vi "Generate Simulated Data.vi"(7 "Type de mode":bool, 8 "error in (no error)":T2 caption="entrée d'erreur (pas d'erreur)", 9 "Péri":tag="Dev1", 10 "Longueur d'onde":dbl, 11 "Type de signal":T1) -> (0 "error out":T2 caption="sortie d'erreur", 2 "Données du graphe":waveform(dbl)[](array[waveform]))   [LabVIEW 2018, in "Acquisition.lvlib"]
doc: "Génère des exemples de waveforms en fonction du type de signal dans l'entrée Configuration du matériel."
uses:
  Acquisition.lvlib
  Signal Type.ctl
  <vilib>/Analysis/baseanly.llb/Mean (DBL).vi
  <vilib>/Analysis/NI_AALBase.lvlib
panel:
  out "Graphe déroulant":dynamicdata(graph)
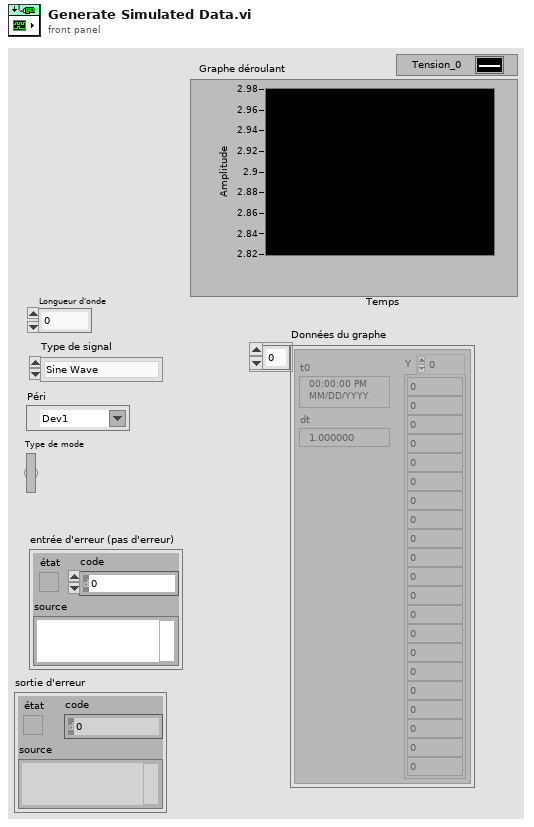
[diagram p1: front panel]
types:
  T1 = typedef "Acquisition.lvlib/Signal Type.ctl" = enum16{"Sine Wave", "Square with Noise", "Signal triangulaire", "Simulation DAQ"}
  T2 = cluster{"état":bool, "code":i32, "source":string}
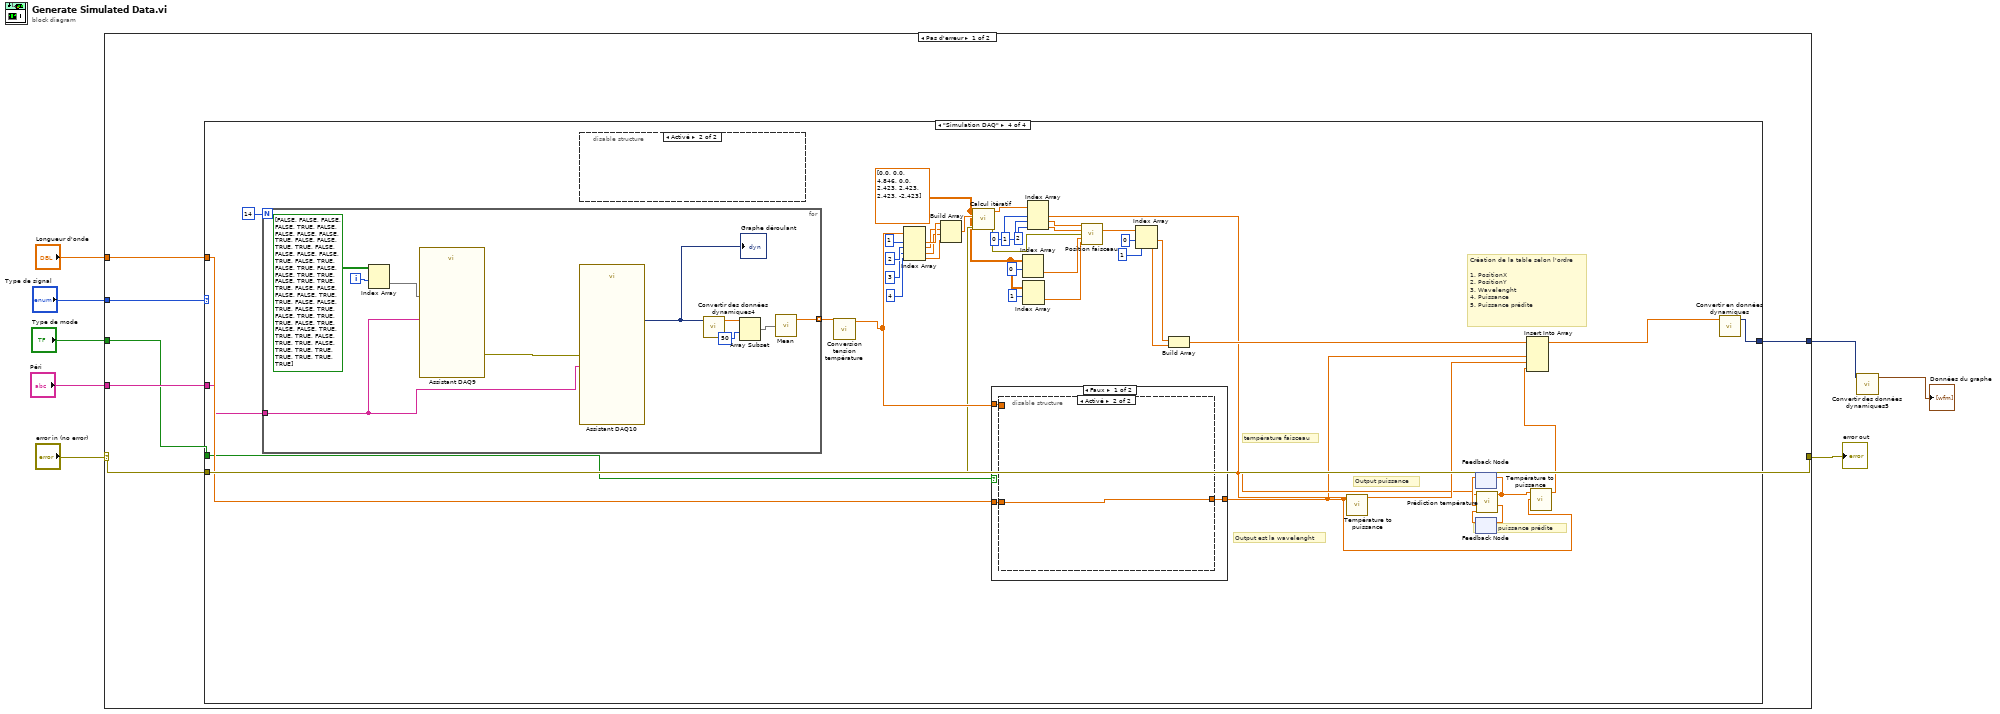
[diagram p0: block diagram]
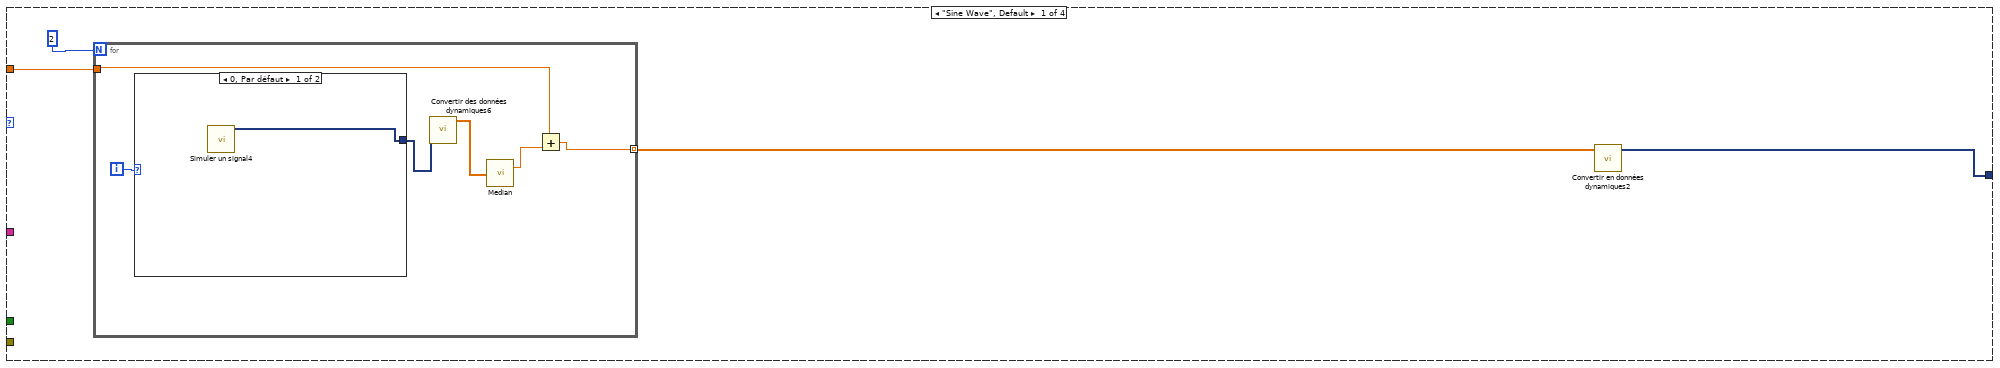
[diagram p2: hidden frame]
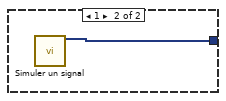
[diagram p3: hidden frame]
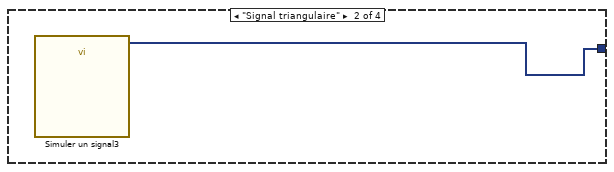
[diagram p4: hidden frame]
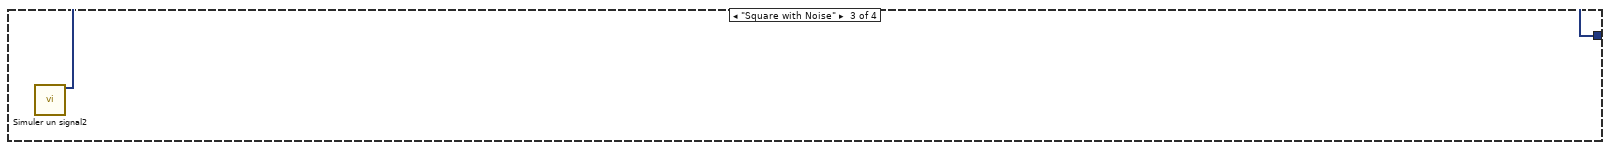
[diagram p5: hidden frame]
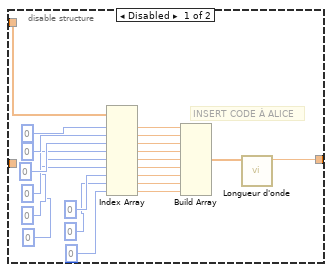
[diagram p6: hidden frame]
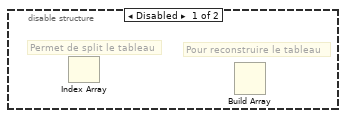
[diagram p8: hidden frame]
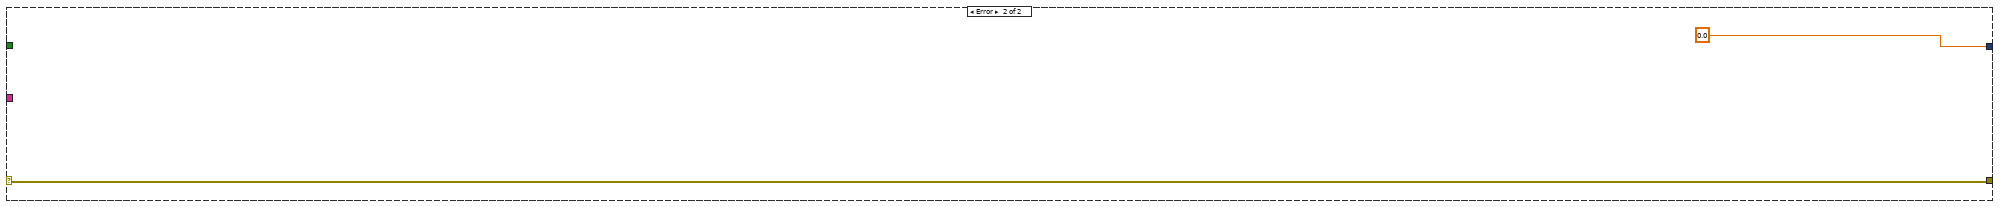
[diagram p9: hidden frame]
diagram:
  n1 = case shown="Pas d'erreur" "error in (no error)" {
    selector: "error in (no error)" -> [w9 w110]
    tunnel: [w9 w110] -> w7
    tunnel: "Type de signal" -> [w14 _]
    tunnel: [w13 0.0] -> w4
    tunnel: "Longueur d'onde" -> [w12 _]
    tunnel: "Péri" -> [w11 _]
    tunnel: "Type de mode" -> [w10 _]
    frame No Error {
      n2 = case shown="\"Simulation DAQ\"" w14 {
        tunnel: [w17 w27 w28 w71] -> w13
        tunnel: w12 -> [w16 _ _ w70]
        tunnel: w11 -> [_ _ _ w69]
        tunnel: w10 -> [_ _ _ w68]
        tunnel: w9 -> [_ _ _ w64]
        frame "Sine Wave", Default {
          n3 = for {
            N: 2 -> [_]
            tunnel: [w20] -> w15 mode=indexing
            tunnel: w16 -> [w19]
            i -> [w24]
            n4 = case shown="0, Par défaut" w24 {
              tunnel: [w25 w26] -> w23
              frame 0, Default {
                n5 = call "Simuler un signal4"() -> ("CC"=w25:dynamicdata)  [unwired: 14 in, 1 out]
              }
              frame 1 {
                n6 = call "Simuler un signal"() -> ("Sinus avec Bruit uniforme"=w26:dynamicdata)  [unwired: 14 in, 1 out]
              }
            }
            n7 = call "Convertir des données dynamiques6"("Dynamic Data Type"=w23) -> ("Array"=w22:dbl[])  [unwired: 3 in]
            n8 = call <vilib>:"Median.vi"("X"=w22) -> ("median"=w21:dbl)  [unwired: 1 out]
            n9 = Add(x=w19, y=w21) -> (x+y=w20:dbl)
          }
          n10 = call "Convertir en données dynamiques2"("Array"=w15) -> ("Dynamic Data Type"=w17:dynamicdata)  [unwired: 3 in]
        }
        frame "Signal triangulaire" {
          n11 = call "Simuler un signal3"() -> ("Triangle"=w27:dynamicdata)  [unwired: 14 in, 1 out]
        }
        frame "Square with Noise" {
          n12 = call "Simuler un signal2"() -> ("Square with Gaussian Noise"=w28:dynamicdata)  [unwired: 14 in, 1 out]
        }
        frame "Simulation DAQ" {
          w60 = dbl[][] [[0.0, 0.0], [4.846, 0.0], [2.423, 2.423], [2.423, -2.423]] ("Position des capteurs")
          # "température faisceau"
          # "Output puissance prédite"
          # "Création de la table selon l'ordre\n\n1. PositionX\n2. PositionY\n3. Wavelenght\n4. Puissance\n5. Puissance prédite"
          # "Output puissance"
          # "Output est la wavelenght"
          n13 = for {
            N: 14 -> [_]
            tunnel: [w100] -> w66 mode=indexing
            tunnel: w69 -> [w99]
            i -> [w106]
            n14 = Index Array(array=bool[][] [[FALSE, FALSE, FALSE, FALSE], [TRUE, FALSE, FALSE, FALSE], [FALSE, TRUE, FALSE, FALSE], [TRUE, TRUE, FALSE, FALSE], [FALSE, FALSE, TRUE, FALSE], [TRUE, FALSE, TRUE, FALSE], [FALSE, TRUE, TRUE, FALSE], [TRUE, TRUE, TRUE, FALSE], [FALSE, FALSE, FALSE, TRUE], [TRUE, FALSE, FALSE, TRUE], [FALSE, TRUE, FALSE, TRUE], [TRUE, TRUE, FALSE, TRUE], [FALSE, FALSE, TRUE, TRUE], [TRUE, FALSE, TRUE, TRUE], [FALSE, TRUE, TRUE, TRUE], [TRUE, TRUE, TRUE, TRUE]], index (row)=w106) -> (element=w105:bool[])  [unwired: 1 in]
            n15 = call "Assistant DAQ9"("data"=w105, "nom du périphérique"=w99) -> ("error out"=w108:errorcluster)  [unwired: 16 in, 1 out]
            n16 = call "Assistant DAQ10"("error in"=w108, "nom du périphérique"=w99) -> ("data"=w104:dynamicdata)  [unwired: 15 in, 2 out]
            "Graphe déroulant" <- w104
            n17 = call "Convertir des données dynamiques4"("Dynamic Data Type"=w104) -> ("Array"=w103:dbl[])  [unwired: 3 in]
            n18 = Array Subset(array=w103, index=50 ("indice")) -> (w101:dbl[])  [unwired: 1 in]
            n19 = call-poly <vilib>:"Mean.vi"("X"=w101) -> ("mean"=w100:dbl)  [unwired: 1 out]
          }
          n20 = disable-structure shown="Activé" {
            frame Disabled {
              # "Pour reconstruire le tableau"
              # "Permet de split le tableau"
              n21 = Index Array() -> ()  [unwired: 2 in, 1 out]
              n22 = Build Array() -> ()  [unwired: 4 in, 1 out]
            }
            frame Enabled {
            }
          }
          n23 = call "Conversion tension température.vi"("Tension In"=w66) -> ("Température Out"=w65:dbl[])  [unwired: 10 in]
          n24 = Index Array(array=w65, index #1=1, index #2=2, index #3=3, index #4=4) -> (element #1=w62:dbl, element #2=w48:dbl, element #3=w47:dbl, element #4=w46:dbl)
          n25 = Build Array(w62, w48, w47, w46) -> (w63:dbl[])
          n26 = call "Calcul itératif.vi"("error in (no error)"=w64, "Température capteur 1-2-3-4-Ambiant"=w63, "Position des capteurs"=w60) -> ("error out"=w37:T2, "DATA - T/R1/R2/R3"=w42:dbl[])  [unwired: 7 in]
          n27 = case shown="Faux" w68 {
            tunnel: [w75 w98] -> w30
            tunnel: w70 -> [w73 w98]
            tunnel: w65 -> [w74 _]
            frame False {
              n28 = disable-structure shown="Activé" {
                disable-tunnel: [w86 w97] -> w75
                disable-tunnel: w74 -> [w76 _]
                disable-tunnel: w73 -> [_ w97]
                frame Disabled {
                  # "INSERT CODE À ALICE"
                  n29 = Index Array(array=w76, index #1=0 ("indice"), index #2=0 ("indice"), index #3=0 ("indice"), index #4=0 ("indice"), index #5=0 ("indice"), index #6=0 ("indice"), index #7=0 ("indice"), index #8=0 ("indice"), index #9=0 ("indice")) -> (element #1=w85:dbl, element #2=w84:dbl, element #3=w83:dbl, element #4=w82:dbl, element #5=w81:dbl, element #6=w80:dbl, element #7=w79:dbl, element #8=w78:dbl, element #9=w77:dbl)
                  n30 = Build Array(w85, w84, w83, w82, w81, w80, w79, w78, w77) -> (w96:dbl[])
                  n31 = call "Longueur d'onde.vi"("T thermistances"=w96) -> ("Longeur d'onde"=w86:dbl)  [unwired: 10 in]
                }
                frame Enabled {
                }
              }
            }
            frame True {
            }
          }
          n32 = Index Array(array=w60, index (row)=0 ("indice (ligne)")) -> (element=w59:dbl[])  [unwired: 1 in]
          n33 = Index Array(array=w60, index (row)=1 ("indice (ligne)")) -> (element=w58:dbl[])  [unwired: 1 in]
          n34 = Index Array(array=w42, index #1=0, index #2=1 ("indice"), index #3=2 ("indice")) -> (element #1=w32:dbl, element #2=w41:dbl, element #3=w40:dbl)
          n35 = call "Position faisceau.vi"("R1"=w41, "R2"=w40, "error in (no error)"=w37, "Capteur 1"=w59, "Capteur 2"=w58) -> ("Coord"=w55:dbl[])  [unwired: 9 in, 1 out]
          n36 = Index Array(array=w55, index #1=0 ("indice"), index #2=1 ("indice")) -> (element #1=w52:dbl, element #2=w51:dbl)
          n37 = Build Array(w52, w51) -> (w39:dbl[])
          n38 = call "Température to puissance.vi"("Longueur d'onde"=w30, "Température max"=w32) -> ("Puissance"=w38:dbl)  [unwired: 9 in]
          n39 = feedback #1() -> (w34:dbl)  [unwired: 1 in]
          n40 = feedback #2() -> (w35:dbl)  [unwired: 1 in]
          n41 = call "Prédiction température.vi"("Temps -2"=w35, "Temps -1"=w34, "Temps 0"=w32) -> ("Temps-1"=w33:dbl, "Temps pred"=w31:dbl)  [unwired: 7 in]
          n42 = feedback-in #1(w31) -> ()
          n43 = feedback-in #2(w33) -> ()
          n44 = call "Température to puissance.vi"("Longueur d'onde"=w30, "Température max"=w31) -> ("Puissance"=w29:dbl)  [unwired: 9 in]
          n45 = Insert Into Array(array=w39, new element #1=w30, new element #2=w38, new element #3=w29) -> (w67:dbl[])  [unwired: 1 in]
          n46 = call "Convertir en données dynamiques"("Array"=w67) -> ("Dynamic Data Type"=w71:dynamicdata)  [unwired: 3 in]
        }
      }
    }
    frame Error {
    }
  }
  "error out" <- w7
  n47 = call "Convertir des données dynamiques5"("Dynamic Data Type"=w4) -> ("Array of Waveform"=→"Données du graphe":waveform(dbl)[])  [unwired: 3 in]
